vi "DELETE.vi"(0 "client handle":T4, 1 "output file":path=path "", 2 "Error code options":T3={"1xx (info)"=FALSE, "2xx (success)"=FALSE, "3xx (redirect)"=FALSE, "4xx (client error)"=TRUE, "5xx (server error)"=TRUE, "Other"=TRUE}, 3 "BlueLogParent in":refnum<class "BlueLogParent_OpenSource.lvclass">, 5 "url":string, 11 "error in (no error)":errorcluster, 12 "timeout (10000)":i32=10000) -> (4 "client handle out":T4, 6 "Header Values":T1[](array[typedef]), 8 "body":string, 10 "HTTP response code":T2, 15 "error out":errorcluster)   [LabVIEW 2020, in "Blue Easy HTTP OpenSource.lvlib"]
doc: "Sends a Web request to delete resources on a server, Web page, or Web service. This VI uses the DELETE HTTP method. The server accepting the request from the DELETE VI must be setup to delete resources solely based upon receiving a DELETE Web request at the specified URL. Refer to the World Wide Web Consortium Web site at www.w3.org for more information about HTTP method definitions, including the DELETE method.\n\nYou can assign a client handle to add authentication credentials, HTTP headers, or a cookie to Web requests made by the DELETE VI. Use the OpenHandle VI to open a client handle and establish credentials. Use the AddHeader VI to add header lines to Web requests made by the DELETE VI."
uses:
  Blue Easy HTTP OpenSource.lvlib
  <vilib>/httpClient/ClientHandle.ctl
  HTTP error on codes.ctl
  HTTP response code.ctl
  HTTP Header.ctl
  <userlib>/Blue Origin/BlueLogParent_OpenSource/BlueLogParentClass/BlueLogParent_OpenSource.lvclass
  Interpret Header.vi
  <vilib>/dlg_ctls.llb/Space Constant.vi
  <vilib>/Utility/error.llb/Trim Whitespace.vi
  <vilib>/Utility/error.llb/Error Cluster From Error Code.vi
  <vilib>/httpClient/LabVIEWHTTPClient.lvlib
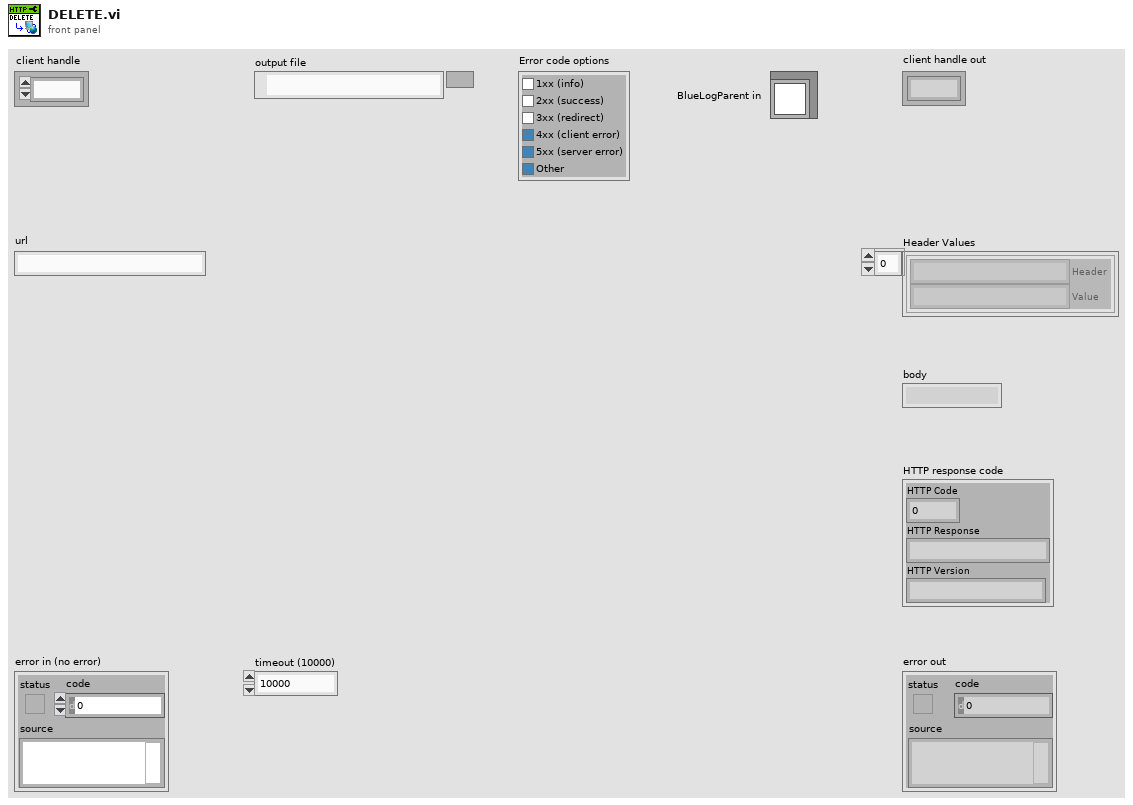
[diagram p1: front panel]
types:
  T1 = typedef "Blue Easy HTTP OpenSource.lvlib/HTTP Header.ctl" = cluster{"Header":string, "Value":string}
  T2 = typedef "Blue Easy HTTP OpenSource.lvlib/HTTP response code.ctl" = cluster{"HTTP Code":u16, "HTTP Response":string, "HTTP Version":string}
  T3 = typedef "Blue Easy HTTP OpenSource.lvlib/HTTP error on codes.ctl" = cluster{"1xx (info)":bool, "2xx (success)":bool, "3xx (redirect)":bool, "4xx (client error)":bool, "5xx (server error)":bool, "Other":bool}
  T4 = typedef "LabVIEWHTTPClient.lvlib/ClientHandle.ctl" = refnum<k1>
  T5 = typedef "BlueLogParent_OpenSource.lvclass/BlueLogParentLevel.ctl" = enum16{"DEBUG", "INFO", "WARNING", "ERROR", "CRITICAL"}
  T6 = typedef "BlueLogParent_OpenSource.lvclass/BlueLogParentOptions.ctl" = cluster{"timestamp (now)":dbl, "Call chain (here)":string, "Count (1)":u16, "Font (override)":T7, "Add row separator? (T)":bool}
  T7 = typedef "BlueLogParent_OpenSource.lvclass/BlueLogParentFont.ctl" = cluster{"Font Name":string, "Size":u16, "Bold":bool, "Italic":bool, "Underline":bool, "Strikeout":bool, "Color":u32}
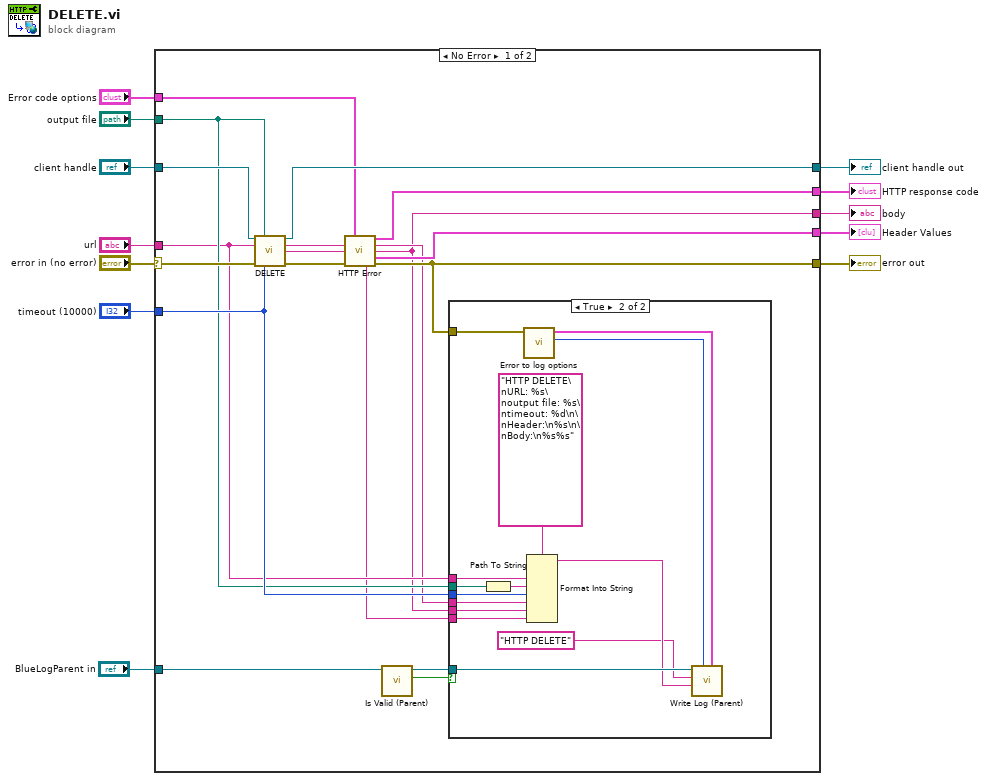
[diagram p0: block diagram]
diagram:
  n1 = case shown="No Error" "error in (no error)" {
    selector: "error in (no error)" -> [w31 w47]
    tunnel: [w19 w47] -> w12
    tunnel: "timeout (10000)" -> [w24 _]
    tunnel: "url" -> [w22 _]
    tunnel: "client handle" -> [w30 w46]
    tunnel: "output file" -> [w23 _]
    tunnel: [w29 w46] -> w6
    tunnel: "Error code options" -> [w27 _]
    tunnel: [w26 _] -> w4
    tunnel: [w17 _] -> w3
    tunnel: [w25 _] -> w2
    tunnel: "BlueLogParent in" -> [w13 _]
    frame No Error {
      n2 = call <vilib>:"DELETE.vi"("client handle"=w30, "output file"=w23, "url"=w22, "error in (no error)"=w31, "timeout (10000)"=w24) -> ("client handle out"=w29:T4, "headers"=w21:string, "body"=w20:string, "error out"=w28:errorcluster)  [unwired: 7 in]
      n3 = call "HTTP Error.vi"("Error code options"=w27, "Header"=w21, "body"=w20, "error in (no error)"=w28) -> ("HTTP response code"=w26:T2, "Header (dup)"=w18:string, "body (dup)"=w17:string, "Header Values"=w25:T1[], "Error log"=w16:string, "error out"=w19:errorcluster)  [unwired: 6 in]
      n4 = call-dynamic "Is Valid (Parent).vi"("BlueLogParent in"=w13) -> ("Is Valid?"=w14:bool, "BlueLogParent out"=w15:refnum<class "BlueLogParent_OpenSource.lvclass">)  [unwired: 8 in, 1 out]
      n5 = case shown="True" w14 {
        tunnel: w19 -> [_ w37]
        tunnel: w22 -> [_ w44]
        tunnel: w23 -> [_ w43]
        tunnel: w24 -> [_ w41]
        tunnel: w17 -> [_ w40]
        tunnel: w18 -> [_ w39]
        tunnel: w15 -> [_ w38]
        tunnel: w16 -> [_ w32]
        frame False {
        }
        frame True {
          n6 = Path To String(path=w43) -> (string=w42:string)
          n7 = call "Error to log options.vi"("error in (no error)"=w37) -> ("Logging level"=w35:T5, "Options"=w36:T6)  [unwired: 9 in]
          n8 = Format Into String(format string="HTTP DELETE\nURL: %s\noutput file: %s\ntimeout: %d\n\nHeader:\n%s\n\nBody:\n%s%s", w44, w42, w41, w39, w40, w32) -> (resulting string=w34:string)  [unwired: 2 in, 1 out]
          n9 = call-dynamic "Write Log (Parent).vi"("Options"=w36, "Logging level (INFO)"=w35, "Message"=w34, "Message Title"="HTTP DELETE" ("Unique ID"), "BlueLogParent in"=w38) -> ()  [unwired: 5 in, 2 out]
        }
      }
    }
    frame Error {
    }
  }
  "error out" <- w12
  "client handle out" <- w6
  "HTTP response code" <- w4
  "body" <- w3
  "Header Values" <- w2
